vi "AFM_Litho_Plugin.IV.IVStatus--Local.vi"(6 "timeout in ms (-1)":i32, 8 "error in (no error)":errorcluster, 11 "MeasurementSMO":refnum<class "AFM_Litho_Plugin.IV.lvclass">) -> (0 "error out":errorcluster, 2 "Running?":bool, 3 "MeasurementSMO out":refnum<class "AFM_Litho_Plugin.IV.lvclass">)   [LabVIEW 2019, in "AFM_Litho_Plugin.IV.lvclass"]
doc: "---------------------------------------------------------------\nJKI State Machine Objects™\nhttp://jki.net/state-machine-objects/\nCopyright (C) 2005-2015, JKI <info@jki.net>\nALL RIGHTS RESERVEDJKI State Machine Objects (SMO) 1.0.0.4\nJKI - JKI\nCopyright (c) 2015, JKI"
uses:
  AFM_Litho_Plugin.IV.lvclass
  Typedefs/PrivateEvents--AFM_Litho_Plugin.IV.IV Status--Local.ctl
  AFM_Litho_Plugin.IV.lvclass/AFM_Litho_Plugin.IV.ctl
panel:
  # "For instructions on how to use the JKI State Machine Objects, examples and video tutorials, visit:\nhttp://jki.net/state-machine-objects/\n\nJKI State Machine Objects™\nhttp://jki.net/state-machine-objects/\nCopyright (C) 2005-2015, JKI <info@jki.net>\nALL RIGHTS RESERVED"
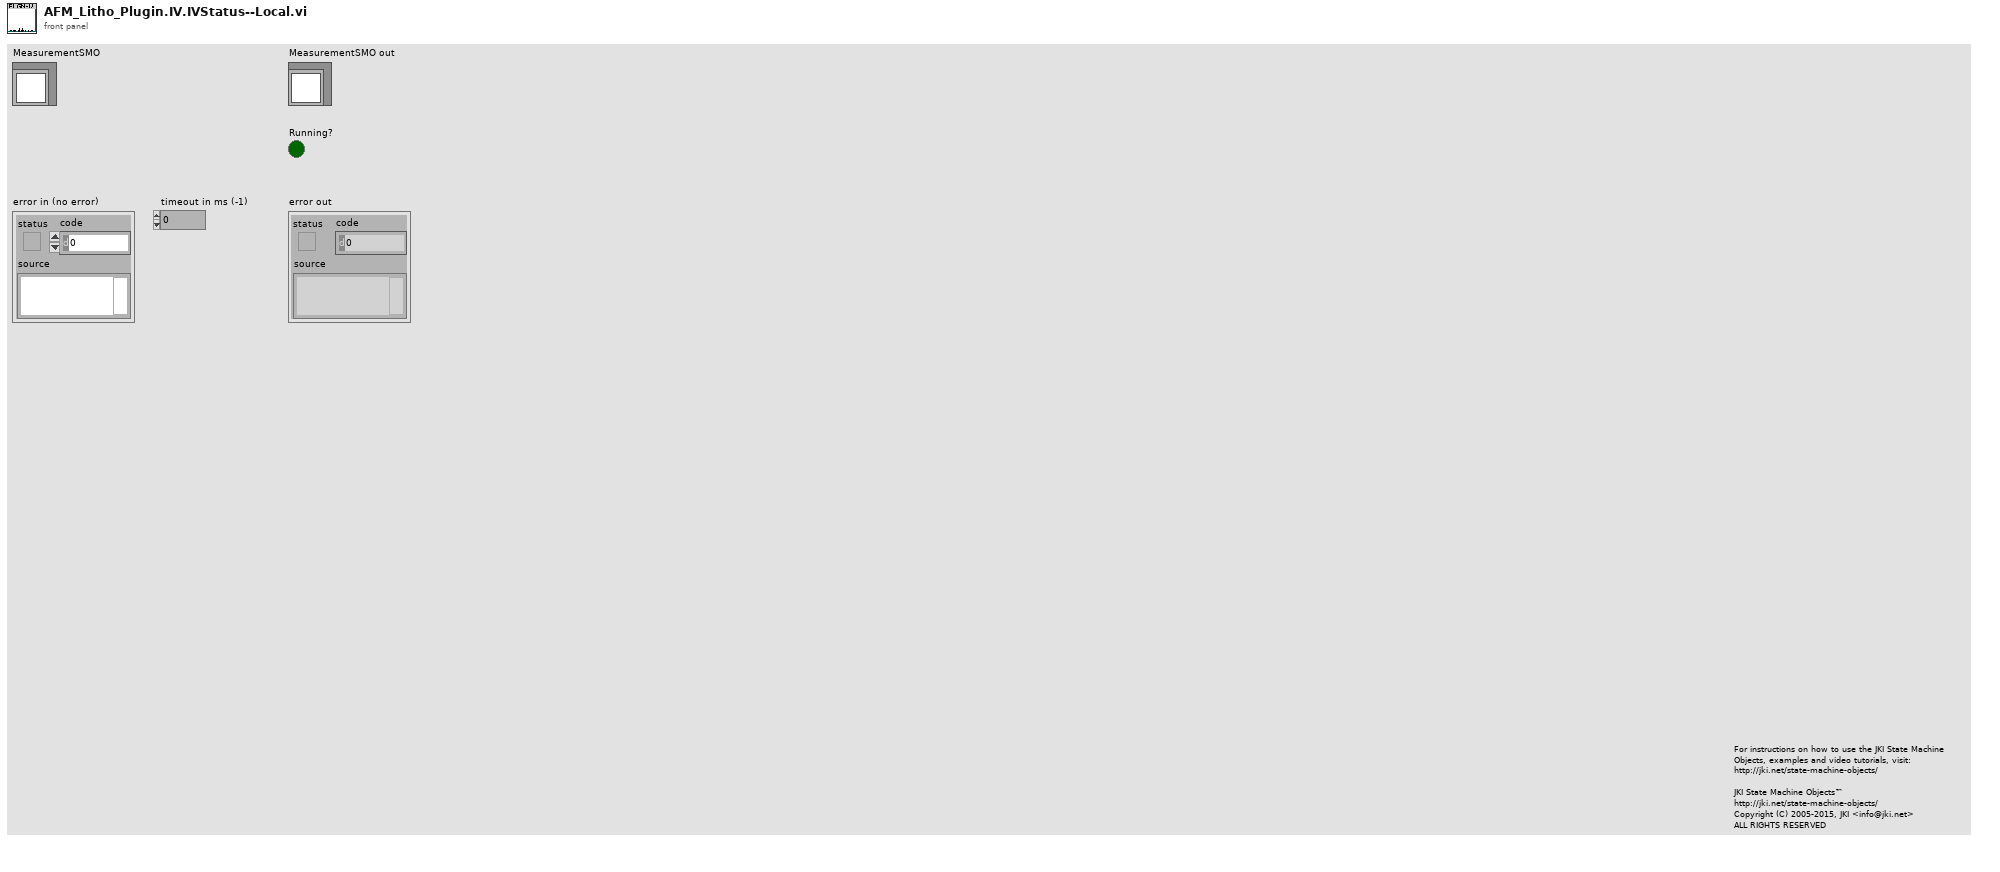
[diagram p1: front panel]
types:
  T1 = typedef "AFM_Litho_Plugin.IV.lvclass/PrivateEvents--AFM_Litho_Plugin.IV.IV Status--Local.ctl" = cluster{"Return":refnum<notifier>}
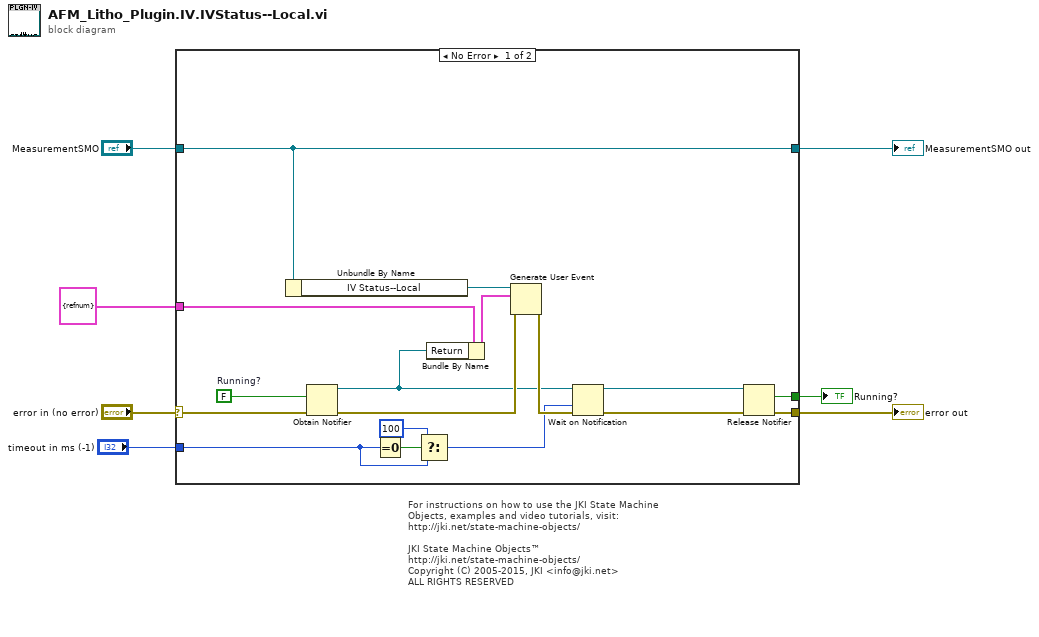
[diagram p0: block diagram]
diagram:
  # "For instructions on how to use the JKI State Machine Objects, examples and video tutorials, visit:\nhttp://jki.net/state-machine-objects/\n\nJKI State Machine Objects™\nhttp://jki.net/state-machine-objects/\nCopyright (C) 2005-2015, JKI <info@jki.net>\nALL RIGHTS RESERVED"
  n1 = case shown="No Error" "error in (no error)" {
    selector: "error in (no error)" -> [w21 w26]
    tunnel: [w19 w26] -> w6
    tunnel: [w23 w25] -> w7
    tunnel: "MeasurementSMO" -> [w23 w25]
    tunnel: T1 {"Return"=refnum} ("IV Status--Local") -> [w13 _]
    tunnel: [w18 _] -> w2
    tunnel: "timeout in ms (-1)" -> [w8 _]
    frame No Error {
      w22 = FALSE  # Running?
      n2 = Unbundle By Name(w23) -> ("IV Status--Local"=w24:refnum<user-event>)
      n3 = Obtain Notifier(notification data type=w22, error in (no error)=w21) -> (notifier out=w12:refnum<notifier>, error out=w16:errorcluster)  [unwired: 2 in, 1 out]
      n4 = Equal To 0?(x=w8) -> (x = 0?=w11:bool)
      n5 = Select(t=100, s=w11, f=w8) -> (s? t:f=w9:i32)
      n6 = Bundle By Name(cluster=w13, "Return"=w12) -> (w14:T1)
      n7 = Generate User Event(user event=w24, event data cluster=w14, error in=w16) -> (error out=w15:errorcluster)  [unwired: 1 in, 1 out]
      n8 = Wait on Notification(notifier=w12, timeout in ms (-1)=w9, error in (no error)=w15) -> (notifier out=w20:refnum<notifier>, error out=w17:errorcluster)  [unwired: 1 in, 2 out]
      n9 = Release Notifier(notifier=w20, error in (no error)=w17) -> (last notification=w18:bool, error out=w19:errorcluster)  [unwired: 1 in, 1 out]
    }
    frame Error {
    }
  }
  "error out" <- w6
  "MeasurementSMO out" <- w7
  "Running?" <- w2
